vi "DAQNavi Write (Analog Wfm 1Chan 1Samp).vi"(8 "error in (no error)":errorcluster, 9 "timeout":dbl=10.0, 10 "Waveform":waveform(dbl), 11 "task in":i32) -> (0 "error out":errorcluster, 2 "number of samples written per channel":u32, 3 "task out":i32)   [LabVIEW 2020]
uses:
  DAQNavi_LV.dll
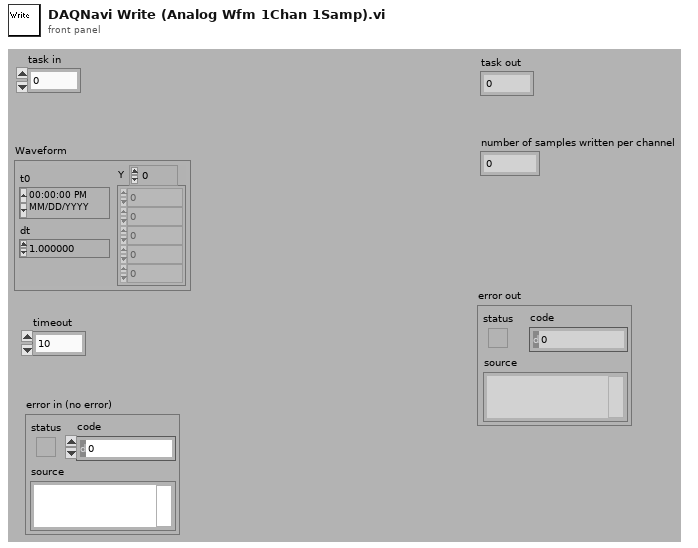
[diagram p1: front panel]
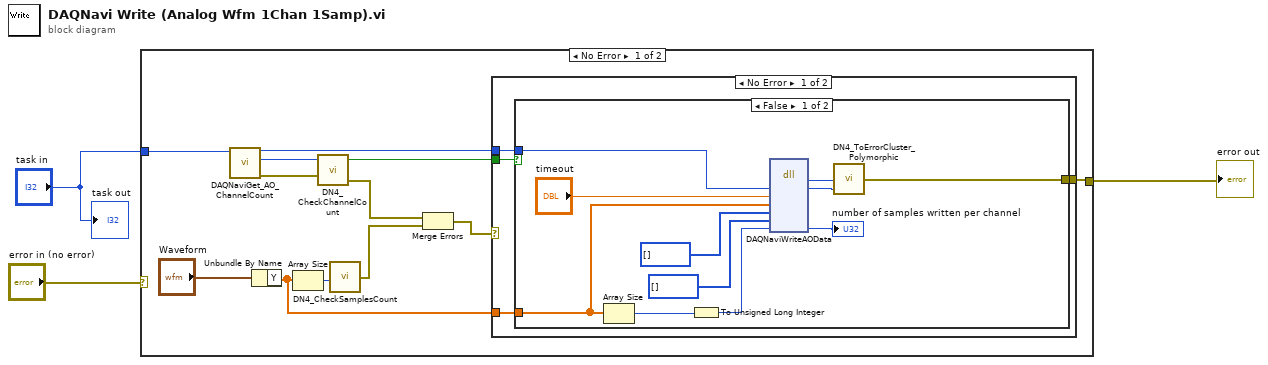
[diagram p0: block diagram]
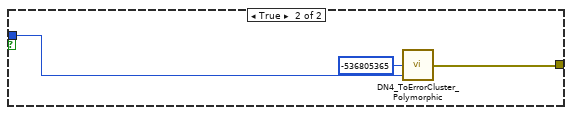
[diagram p2: hidden frame]
diagram:
  n1 = case shown="No Error" "error in (no error)" {
    selector: "error in (no error)" -> [_ w35]
    tunnel: [w14 w35] -> w2
    tunnel: "task in" -> [w15 _]
    frame No Error {
      n2 = call "DAQNaviGet_AO_ChannelCount.vi"("task in"=w15) -> ("error out"=w11:errorcluster, "channel count"=w12:i32, "task out"=w10:i32)  [unwired: 1 in, 7 out]
      n3 = Unbundle By Name("Waveform") -> ("Y"=w5:dbl[])
      n4 = Array Size(array=w5) -> (size(s)=w6:i32)
      n5 = call "DN4_CheckChannelCount.vi"("error out"=w11, "channel count"=w12) -> ("error IO"=w8:errorcluster, "greater than 1?"=w9:bool)  [unwired: 2 out]
      n6 = call "DN4_CheckSamplesCount.vi"("samples count"=w6) -> ("error out"=w7:errorcluster)
      n7 = Merge Errors(w8, w7) -> (w13:errorcluster)
      n8 = case shown="No Error" w13 {
        selector: w13 -> [_ w34]
        tunnel: w9 -> [w19 _]
        tunnel: w10 -> [w18 _]
        tunnel: [w17 w34] -> w14
        tunnel: w5 -> [w16 _]
        frame No Error {
          n9 = case shown="False" w19 {
            tunnel: [w24 w32] -> w17
            tunnel: w18 -> [w30 w31]
            tunnel: w16 -> [w23 _]
            frame False {
              n10 = Array Size(array=w23) -> (size(s)=w22:i32)
              n11 = To Unsigned Long Integer(number=w22) -> (unsigned 32bit integer=w21:u32)
              n12 = dll-call lib="DAQNavi_LV.dll" fn="DAQNaviWriteAOData"("taskID"=w30, "timeout"="timeout", "scaledData"=w23, "rawData16"=u16[] [], "rawData32"=u32[] [], "samples"=w21) -> ("return type"=w25:i32, "taskID"=w20:i32, "samples"=→"number of samples written per channel":u32)  [unwired: 5 in, 4 out]
              n13 = call "DN4_ToErrorCluster_Polymorphic.vi"("task id"=w20, "error code"=w25) -> ("error out"=w24:errorcluster)  [unwired: 3 out]
            }
            frame True {
              n14 = call "DN4_ToErrorCluster_Polymorphic.vi"("task id"=w31, "error code"=-536805365) -> ("error out"=w32:errorcluster)  [unwired: 3 out]
            }
          }
        }
        frame Error {
        }
      }
    }
    frame Error {
    }
  }
  "error out" <- w2
  "task out" <- "task in"
